vi "PointROIToBoxROI.vi"(6 "Scan Settings":T3, 8 "Number of Boxes":i32, 9 "Box Offset Z (pixels)":i32, 10 "Box Size (pixels)":i32, 11 "PT ROIs":T2(array[cluster])) -> (2 "Number of Motion Volumes":i32, 3 "BOX ROIs":T2(array[cluster]))   [LabVIEW 2014]
panel:
  in  "Cluster":T1
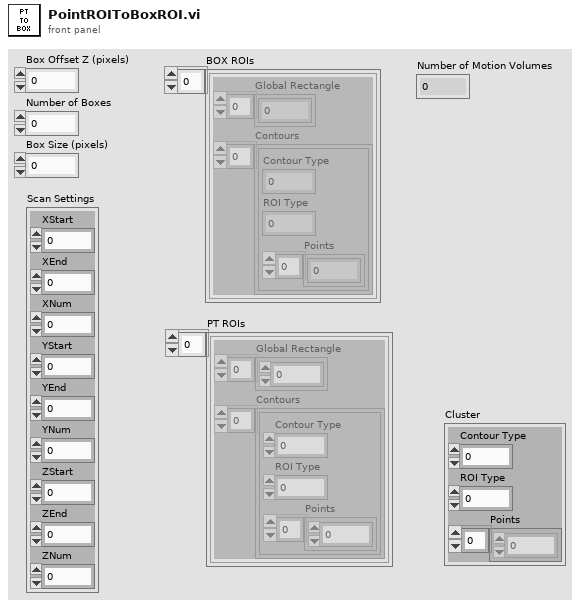
[diagram p1: front panel]
types:
  T1 = cluster{"Contour Type":u32, "ROI Type":u32, "Points":i32[]}
  T2 = cluster{"Global Rectangle":i32[], "Contours":cluster{"Contour Type":u32, "ROI Type":u32, "Points":i32[]}[]}[]
  T3 = cluster{"XStart":i32, "XEnd":i32, "XNum":i32, "YStart":i32, "YEnd":i32, "YNum":i32, "ZStart":i32, "ZEnd":i32, "ZNum":i32}
  T4 = cluster{"Global Rectangle":i32[], "Contours":cluster{"Contour Type":u32, "ROI Type":u32, "Points":i32[]}[]}
  T5 = cluster{"Contour Type":u32, "ROI Type":u32, "Points":i32[]}[]
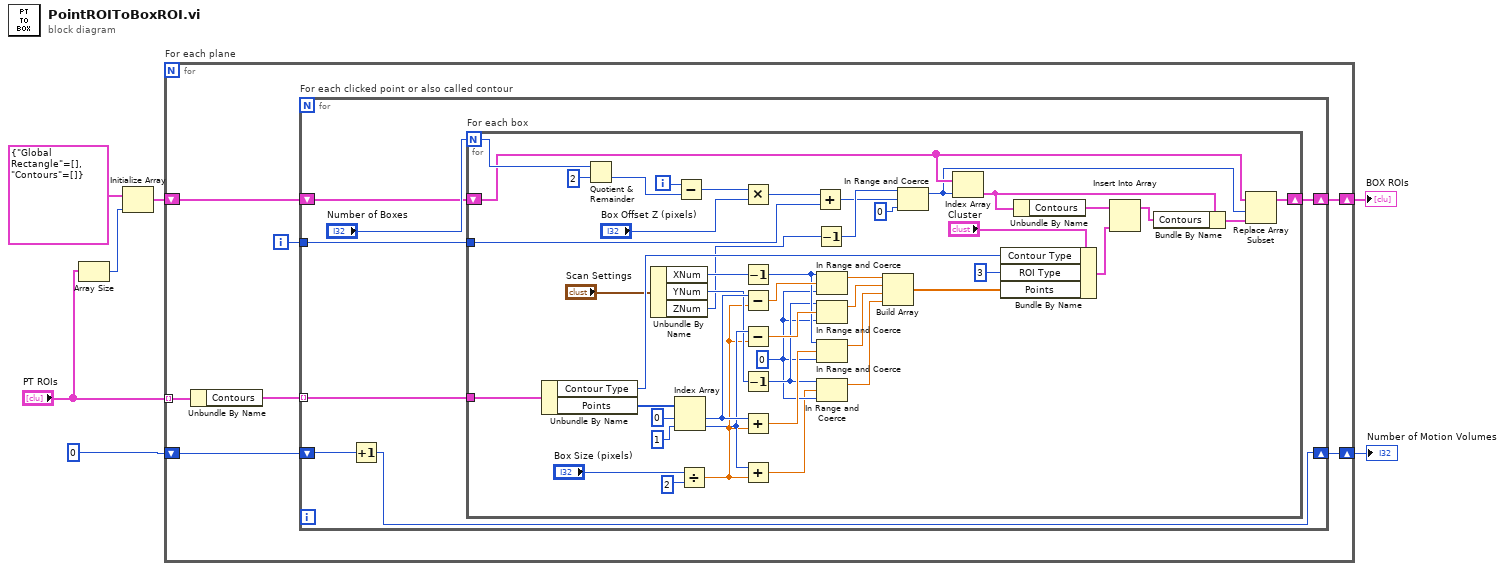
[diagram p0: block diagram]
diagram:
  n1 = Array Size(array="PT ROIs") -> (size(s)=w4:i32)
  n2 = Initialize Array(T4 {"Global Rectangle"=[], "Contours"=[]} ("ROI"), w4) -> (w6:T2)
  n3 = for "For each plane" {
    shift-right: [w11] -> w3
    shift-left: w6 -> [w13]
    tunnel: "PT ROIs" -> [w14] mode=indexing
    shift-right: [w8] -> w1
    shift-left: 0 -> [w9]
    i -> [w10]
    n4 = Unbundle By Name(w14) -> ("Contours"=w12:T5)
    n5 = for "For each clicked point or also called contour" {
      tunnel: w12 -> [w20] mode=indexing
      shift-right: [w18] -> w11
      shift-left: w13 -> [w19]
      tunnel: w10 -> [w17]
      shift-right: [w15] -> w8
      shift-left: w9 -> [w16]
      n6 = Increment(x=w16) -> (x+1=w15:i32)
      n7 = for "For each box" {
        N: "Number of Boxes" -> [w62]
        tunnel: w20 -> [w58]
        shift-right: [w42] -> w18
        shift-left: w19 -> [w44]
        tunnel: w17 -> [w40]
        i -> [w63]
        w28 = 0 ("y")
        n8 = Unbundle By Name(w58) -> ("Contour Type"=w55:u32, "Points"=w56:i32[])
        n9 = Quotient & Remainder(x=w62, y=2) -> (floor(x/y)=w64:i32)  [unwired: 1 out]
        n10 = Unbundle By Name("Scan Settings") -> ("XNum"=w51:i32, "YNum"=w50:i32, "ZNum"=w49:i32)
        n11 = Index Array(array=w56, index #1=0 ("index"), index #2=1 ("index")) -> (element #1=w66:i32, element #2=w65:i32)
        n12 = Subtract(x=w63, y=w64) -> (x-y=w59:i32)
        n13 = Divide(x="Box Size (pixels)", y=2) -> (x/y=w39:dbl)
        n14 = Multiply(x=w59, y="Box Offset Z (pixels)") -> (x*y=w41:i32)
        n15 = Decrement(x=w51) -> (x-1=w32:i32)
        n16 = Subtract(x=w66, y=w39) -> (x-y=w36:dbl)
        n17 = Subtract(x=w65, y=w39) -> (x-y=w34:dbl)
        n18 = Decrement(x=w50) -> (x-1=w29:i32)
        n19 = Add(x=w66, y=w39) -> (x+y=w31:dbl)
        n20 = Add(x=w65, y=w39) -> (x+y=w27:dbl)
        n21 = Add(x=w41, y=w40) -> (x+y=w24:i32)
        n22 = Decrement(x=w49) -> (x-1=w25:i32)
        n23 = In Range and Coerce(upper limit=w32, x=w36, lower limit=w28) -> (coerced(x)=w35:dbl)  [unwired: 1 out]
        n24 = In Range and Coerce(upper limit=w29, x=w34, lower limit=w28) -> (coerced(x)=w33:dbl)  [unwired: 1 out]
        n25 = In Range and Coerce(upper limit=w32, x=w31, lower limit=w28) -> (coerced(x)=w30:dbl)  [unwired: 1 out]
        n26 = In Range and Coerce(upper limit=w29, x=w27, lower limit=w28) -> (coerced(x)=w26:dbl)  [unwired: 1 out]
        n27 = Build Array(w35, w33, w30, w26) -> (w53:dbl[])
        n28 = In Range and Coerce(upper limit=w25, x=w24, lower limit=0 ("y")) -> (coerced(x)=w22:i32)  [unwired: 1 out]
        n29 = Index Array(array=w44, index=w22) -> (element=w46:T4)
        n30 = Bundle By Name(cluster="Cluster", "Contour Type"=w55, "ROI Type"=u32 3, "Points"=w53) -> (w48:T1)
        n31 = Unbundle By Name(w46) -> ("Contours"=w47:T5)
        n32 = Insert Into Array(array=w47, new element=w48) -> (w45:T5)  [unwired: 1 in]
        n33 = Bundle By Name(cluster=w46, "Contours"=w45) -> (w43:T4)
        n34 = Replace Array Subset(array=w44, new element=w43, index=w22) -> (w42:T2)
      }
    }
  }
  "BOX ROIs" <- w3
  "Number of Motion Volumes" <- w1
